vi "DB-初始化.vi"(7 "table-探测器列表名":string="探测器列表", 8 "error in (no error)":errorcluster, 11 "数据库引用":T1) -> (0 "error out":errorcluster, 3 "connection reference out":T1)   [LabVIEW 2017]
uses:
  <vilib>/addons/database/Connection.llb/Conn ObjectReference.ctl
  <vilib>/addons/database/Auxilliary.llb/DB Tools Column Info.ctl
  <vilib>/addons/database/Auxilliary.llb/DB Tools DataTypes.ctl
  <vilib>/addons/database/NI_Database_API.lvlib
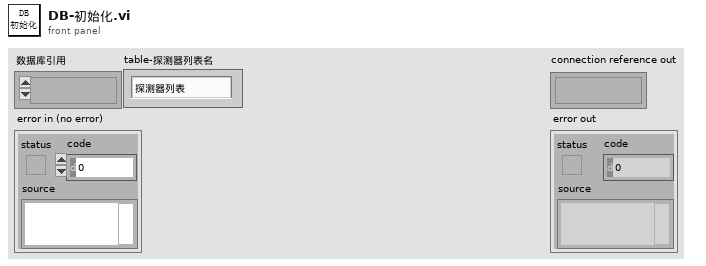
[diagram p1: front panel]
types:
  T1 = typedef "NI_Database_API.lvlib/Conn ObjectReference.ctl" = refnum<k1>
  T2 = typedef "探测器信息.ctl" = cluster{"网络地址":string, "名称":string, "备注":string, "累积剂量":dbl, "累积限值":dbl, "硬件剂量率限值":T3, "剂量率限值1":dbl, "剂量率限值2":dbl, "报警方式":T4}
  T3 = typedef "探头剂量率限值选择.ctl" = enum16{"一级限值", "二级限值"}
  T4 = typedef "报警方式选择.ctl" = enum16{"常报警", "自动静音", "手动静音"}
  T5 = typedef "NI_Database_API.lvlib/DB Tools Column Info.ctl" = cluster{"column name":string, "data type":T6, "size":i32, "allow null?":bool}
  T6 = typedef "NI_Database_API.lvlib/DB Tools DataTypes.ctl" = enum16{"String", "Long (I32)", "Single (SGL)", "Double (DBL)", "Date/Time", "Binary"}
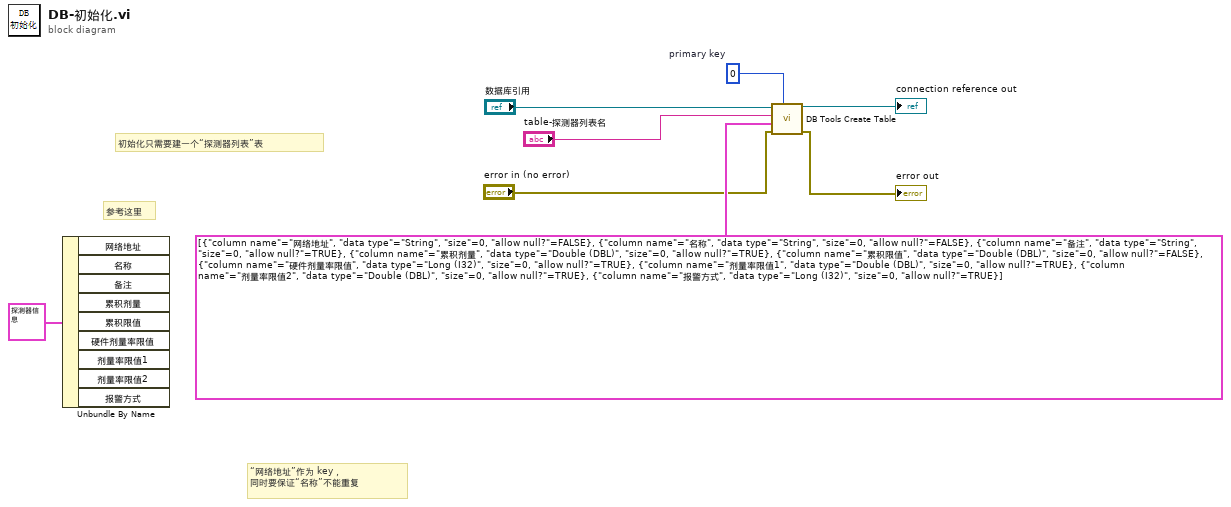
[diagram p0: block diagram]
diagram:
  w8 = 0  # primary key
  # "参考这里"
  # "“网络地址”作为 key，\n同时要保证“名称”不能重复"
  # "初始化只需要建一个“探测器列表”表"
  n1 = Unbundle By Name(T2 {"网络地址"="", "名称"="", "备注"="", "累积剂量"=0.0, "累积限值"=0.0, "硬件剂量率限值"=enum."一级限值", "剂量率限值1"=0.0, "剂量率限值2"=0.0, "报警方式"=enum."常报警"} ("探测器信息")) -> ()  [unwired: 9 out]
  n2 = call <vilib>:"DB Tools Create Table.vi"("primary key (-1)"=w8, "error in (no error)"="error in (no error)", "column information"=T5[] [{"column name"="网络地址", "data type"=enum."String", "size"=0, "allow null?"=FALSE}, {"column name"="名称", "data type"=enum."String", "size"=0, "allow null?"=FALSE}, {"column name"="备注", "data type"=enum."String", "size"=0, "allow null?"=TRUE}, {"column name"="累积剂量", "data type"=enum."Double (DBL)", "size"=0, "allow null?"=TRUE}, {"column name"="累积限值", "data type"=enum."Double (DBL)", "size"=0, "allow null?"=FALSE}, {"column name"="硬件剂量率限值", "data type"=enum."Long (I32)", "size"=0, "allow null?"=TRUE}, {"column name"="剂量率限值1", "data type"=enum."Double (DBL)", "size"=0, "allow null?"=TRUE}, {"column name"="剂量率限值2", "data type"=enum."Double (DBL)", "size"=0, "allow null?"=TRUE}, {"column name"="报警方式", "data type"=enum."Long (I32)", "size"=0, "allow null?"=TRUE}], "table"="table-探测器列表名", "connection reference"="数据库引用") -> ("error out"=→"error out":errorcluster, "connection reference out"=→"connection reference out":T1)  [unwired: 3 in]
